vi "Preset SERIAL NUMBER validator.vi"(8 "error in (no error)":errorcluster, 10 "SERIAL number":string, 11 "VISA resource in":refnum<visa-resource-name>) -> (0 "error out":errorcluster, 3 "VISA resource out":refnum<visa-resource-name>)   [LabVIEW 2025]
uses:
  Preset Number States--enum.ctl
panel:
  # "Set SERIAL number with validation"
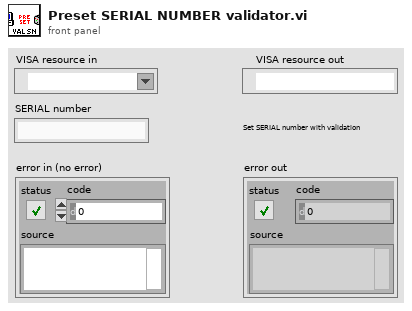
[diagram p1: front panel]
types:
  T1 = typedef "Preset Number States--enum.ctl" = enum16{"Initialize", "Check <=UL", "Check >=LL", "Truncate string", "Send command", "Shutdown"}
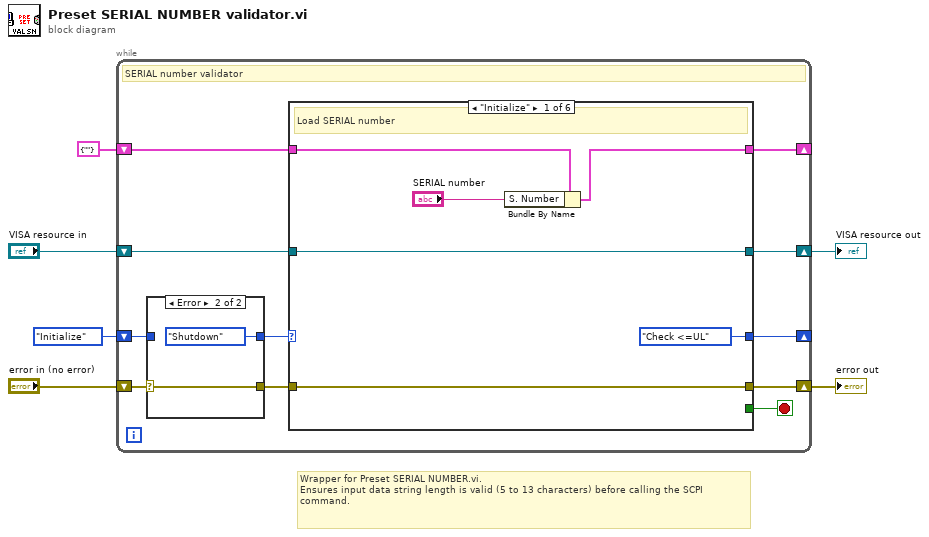
[diagram p0: block diagram]
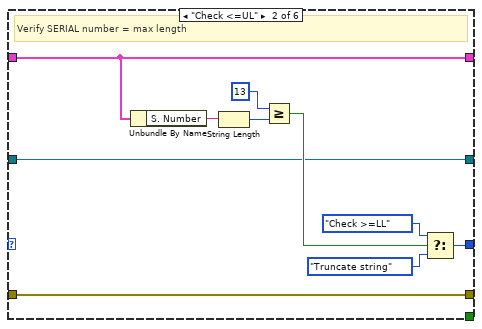
[diagram p3: hidden frame]
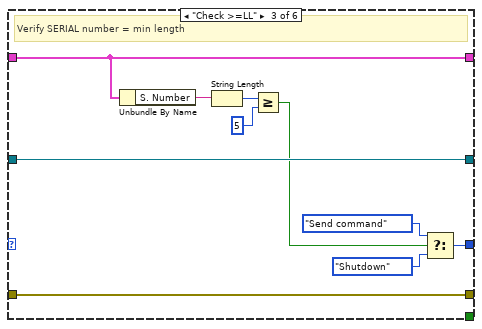
[diagram p4: hidden frame]
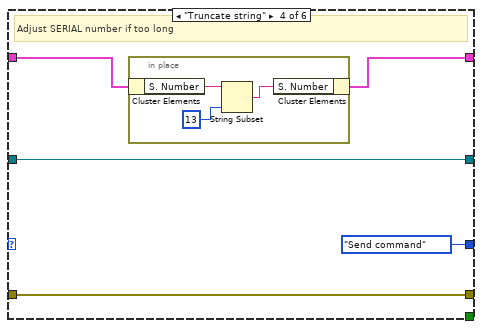
[diagram p5: hidden frame]
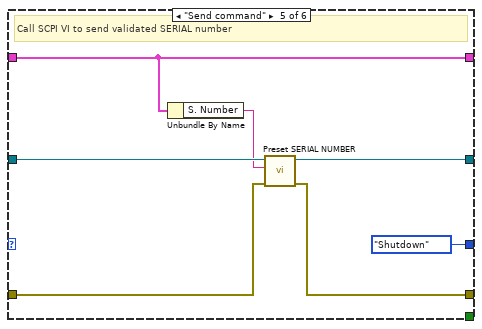
[diagram p6: hidden frame]
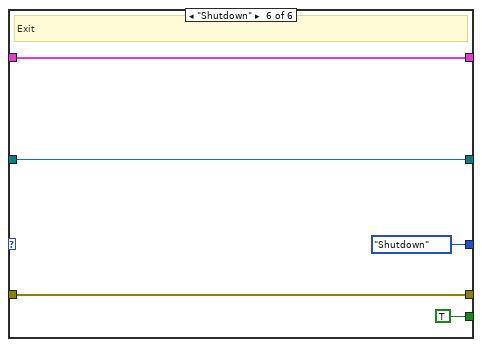
[diagram p7: hidden frame]
diagram:
  # "Wrapper for Preset SERIAL NUMBER.vi.\nEnsures input data string length is valid (5 to 13 characters) before calling the SCPI command."
  n1 = while {
    shift-right: [w14] -> _
    shift-left: Preset_Number_States--enum."Initialize" -> [w13]
    shift-right: [w8] -> _
    shift-left: cluster{"S. Number":string} {"S. Number"=""} -> [w15]
    shift-right: [w9] -> w3
    shift-left: "VISA resource in" -> [w12]
    shift-right: [w10] -> w4
    shift-left: "error in (no error)" -> [w16]
    stop <- w7 stop-if-true
    # "SERIAL number validator"
    n2 = case shown="Error" w16 {
      selector: w16 -> [w19 w20]
      tunnel: [w19 w20] -> w11
      tunnel: [w18 Preset_Number_States--enum."Shutdown"] -> w17
      tunnel: w13 -> [w18 _]
      frame No Error {
      }
      frame Error {
      }
    }
    n3 = case shown="\"Initialize\"" w17 {
      tunnel: w15 -> [w25 w30 w39 w49 w61 w65]
      tunnel: [Preset_Number_States--enum."Check <=UL" w34 w43 Preset_Number_States--enum."Send command" Preset_Number_States--enum."Shutdown" Preset_Number_States--enum."Shutdown"] -> w14
      tunnel: w12 -> [w26 w33 w47 w52 w58 w67]
      tunnel: w11 -> [w27 w32 w46 w51 w60 w66]
      tunnel: [w27 w32 w46 w51 w59 w66] -> w10
      tunnel: [w26 w33 w47 w52 w57 w67] -> w9
      tunnel: [w24 w30 w39 w48 w61 w65] -> w8
      tunnel: [_ _ _ _ _ TRUE] -> w7
      frame "Initialize" {
        # "Load SERIAL number"
        n4 = Bundle By Name(cluster=w25, "S. Number"="SERIAL number") -> (w24:cluster{"S. Number":string})
      }
      frame "Check <=UL" {
        # "Verify SERIAL number = max length"
        n5 = Unbundle By Name(w30) -> ("S. Number"=w29:string)
        n6 = String Length(string=w29) -> (length=w36:i32)
        n7 = Greater Or Equal?(x=13 ("y"), y=w36) -> (x >= y?=w35:bool)
        n8 = Select(t=Preset_Number_States--enum."Check >=LL", s=w35, f=Preset_Number_States--enum."Truncate string") -> (s? t:f=w34:T1)
      }
      frame "Check >=LL" {
        # "Verify SERIAL number = min length"
        n9 = Unbundle By Name(w39) -> ("S. Number"=w38:string)
        n10 = String Length(string=w38) -> (length=w45:i32)
        n11 = Greater Or Equal?(x=w45, y=5) -> (x >= y?=w42:bool)
        n12 = Select(t=Preset_Number_States--enum."Send command" ("f"), s=w42, f=Preset_Number_States--enum."Shutdown") -> (s? t:f=w43:T1)
      }
      frame "Truncate string" {
        # "Adjust SERIAL number if too long"
        n13 = in-place "In Place Element Structure" {
          n14 = in-place-cluster #1 ("Unbundle / Bundle Elements")(w49) -> ("S. Number"=w54:string)
          n15 = String Subset(string=w54, length (rest)=13 ("length (rest)")) -> (substring=w53:string)  [unwired: 1 in]
          n16 = in-place-cluster #1 ("Unbundle / Bundle Elements")("S. Number"=w53) -> (w48:cluster{"S. Number":string})
        }
      }
      frame "Send command" {
        # "Call SCPI VI to send validated SERIAL number"
        n17 = Unbundle By Name(w61) -> ("S. Number"=w56:string)
        n18 = call "Preset SERIAL NUMBER.vi"("error in (no error)"=w60, "SERIAL number"=w56, "VISA Refnum in"=w58) -> ("error out"=w59:errorcluster, "VISA Refnum out"=w57:refnum<visa-resource-name>)  [unwired: 7 in]
      }
      frame "Shutdown" {
        # "Exit"
      }
    }
  }
  "error out" <- w4
  "VISA resource out" <- w3
